vi "CloseFile.vi"(8 "error in (no error)":errorcluster, 11 "FileHandler in":refnum<class "FileHandler.lvclass">) -> (0 "error out":errorcluster)   [LabVIEW 2021, in "FileHandler.lvclass"]
uses:
  FileHandler.lvclass
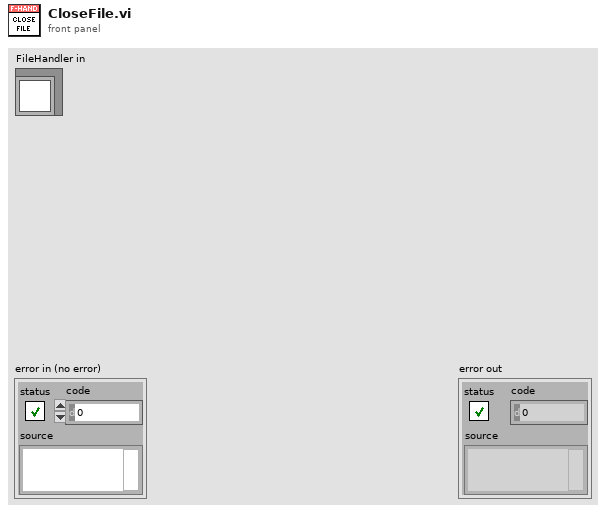
[diagram p1: front panel]
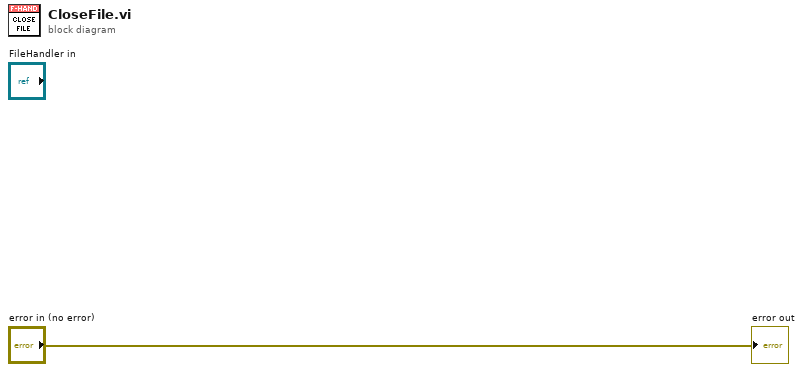
[diagram p0: block diagram]
diagram:
  "error out" <- "error in (no error)"
